vi "getTimeChannelFromXml.vi"(8 "error in (no error)":errorcluster, 10 "Xml":refnum<class "xmlNode.lvclass">, 11 "ScriptEvent in":refnum<class "ScriptEvent.lvclass">) -> (0 "error out":errorcluster, 2 "Xml":refnum<class "xmlNode.lvclass">, 3 "ScriptEvent out":refnum<class "ScriptEvent.lvclass">)   [LabVIEW 2011, in "Tools.lvlib" / "Scripting.lvlib" / "ScriptEvent.lvclass"]
uses:
  ScriptEvent.lvclass
  xmlNode/xmlNode.lvclass
  DatabaseHelpers/Database Objects/Channel/Channel.lvclass
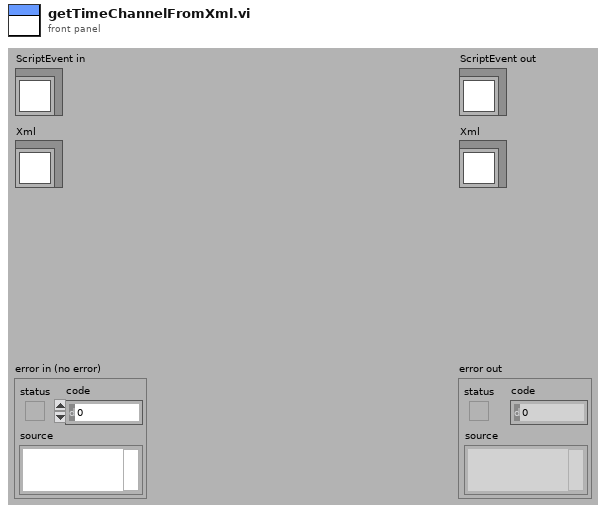
[diagram p1: front panel]
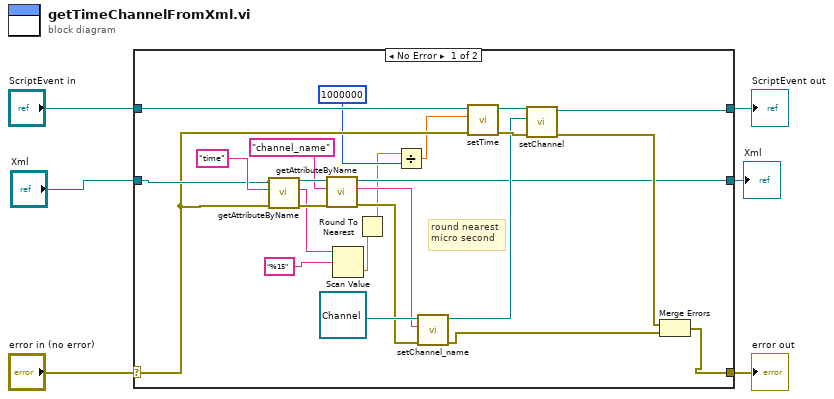
[diagram p0: block diagram]
diagram:
  n1 = case shown="No Error" "error in (no error)" {
    selector: "error in (no error)" -> [w15 w32]
    tunnel: [w14 w32] -> w5
    tunnel: [w18 w31] -> w3
    tunnel: "ScriptEvent in" -> [w20 w31]
    tunnel: "Xml" -> [w19 _]
    tunnel: [w13 _] -> w1
    frame No Error {
      # "round nearest\nmicro second"
      n2 = call-dynamic "getAttributeByName.vi"("error in (no error)"=w15, "AttributeName"="time", "xmlNode in"=w19) -> ("error out"=w29:errorcluster, "attribute string"=w12:string, "xmlNode out"=w28:refnum<class "xmlNode.lvclass">)  [unwired: 6 in]
      n3 = call-dynamic "getAttributeByName.vi"("error in (no error)"=w29, "AttributeName"="channel_name", "xmlNode in"=w28) -> ("error out"=w21:errorcluster, "attribute string"=w25:string, "xmlNode out"=w13:refnum<class "xmlNode.lvclass">)  [unwired: 6 in]
      n4 = Scan Value(string=w12, format string="%15") -> (value=w10:dbl)  [unwired: 1 in, 1 out]
      n5 = Round To Nearest(number=w10) -> (nearest integer value=w7:dbl)
      n6 = Divide(x=w7, y=1000000) -> (x/y=w8:dbl)
      n7 = call "setChannel_name.vi"("error in (no error)"=w21, "channel_name"=w25, "Channel.lvclass in"=refnum<class "Channel.lvclass"> refnum ("Tools.lvlib:DatabaseHelpers.lvlib:Channel.lvclass")) -> ("error out"=w16:errorcluster, "Channel.lvclass out"=w22:refnum<class "Channel.lvclass">)  [unwired: 7 in]
      n8 = call "setTime.vi"("error in (no error)"=w15, "time"=w8, "ScriptEvent.lvclass in"=w20) -> ("error out"=w23:errorcluster, "ScriptEvent.lvclass out"=w24:refnum<class "ScriptEvent.lvclass">)  [unwired: 7 in]
      n9 = call-dynamic "setChannel.vi"("error in (no error)"=w23, "Channel.lvclass"=w22, "ScriptEvent.lvclass in"=w24) -> ("error out"=w17:errorcluster, "ScriptEvent.lvclass out"=w18:refnum<class "ScriptEvent.lvclass">)  [unwired: 7 in]
      n10 = Merge Errors(w17, w16) -> (w14:errorcluster)
    }
    frame Error {
    }
  }
  "error out" <- w5
  "ScriptEvent out" <- w3
  "Xml" <- w1
